vi "Umgebungsdruck beruecksichtigen.vi"(7 "CalGas":bool, 10 "Umgebungsdruck":sgl) -> (2 "Druck Sollwert":sgl)   [LabVIEW 2020, in "Regler.lvlib" / "Druckregler.lvlib"]
uses:
  Druckregler.lvlib
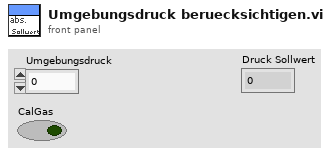
[diagram p1: front panel]
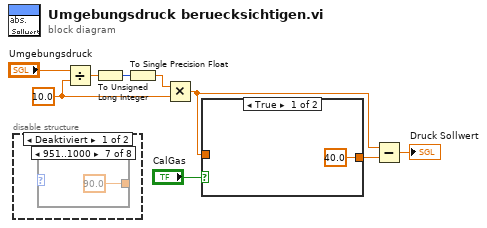
[diagram p0: block diagram]
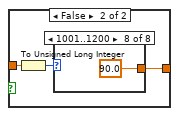
[diagram p2: hidden frame]
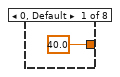
[diagram p3: hidden frame]
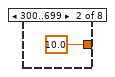
[diagram p4: hidden frame]
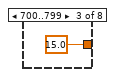
[diagram p5: hidden frame]
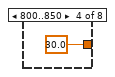
[diagram p6: hidden frame]
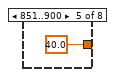
[diagram p7: hidden frame]
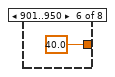
[diagram p8: hidden frame]
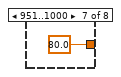
[diagram p9: hidden frame]
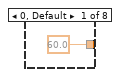
[diagram p10: hidden frame]
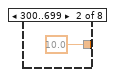
[diagram p11: hidden frame]
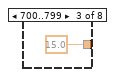
[diagram p12: hidden frame]
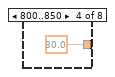
[diagram p13: hidden frame]
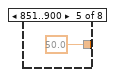
[diagram p14: hidden frame]
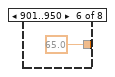
[diagram p15: hidden frame]
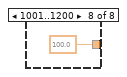
[diagram p16: hidden frame]
diagram:
  w5 = sgl 10.0 ("y")
  n1 = disable-structure shown="Deaktiviert" {
    frame Disabled {
      n2 = case shown="951..1000" {
        selector: _ -> [_ _ _ _ _ _ _ _]
        tunnel: [sgl 60.0 ("y") sgl 10.0 ("y") sgl 15.0 ("y") sgl 30.0 ("y") sgl 50.0 ("y") sgl 65.0 ("y") sgl 90.0 ("y") sgl 100.0 ("y")] -> _
        frame 0, Default {
        }
        frame 300..699 {
        }
        frame 700..799 {
        }
        frame 800..850 {
        }
        frame 851..900 {
        }
        frame 901..950 {
        }
        frame 951..1000 {
        }
        frame 1001..1200 {
        }
      }
    }
    frame Enabled {
    }
  }
  n3 = Divide(x="Umgebungsdruck", y=w5) -> (x/y=w8:sgl)
  n4 = To Unsigned Long Integer(number=w8) -> (unsigned 32bit integer=w7:u32)
  n5 = To Single Precision Float(number=w7) -> (single precision float=w6:sgl)
  n6 = Multiply(x=w6, y=w5) -> (x*y=w2:sgl)
  n7 = case shown="True" "CalGas" {
    tunnel: [sgl 40.0 ("y") w21] -> w9
    tunnel: w2 -> [_ w19]
    frame True {
    }
    frame False {
      n8 = To Unsigned Long Integer(number=w19) -> (unsigned 32bit integer=w20:u32)
      n9 = case shown="1001..1200" w20 {
        tunnel: [sgl 40.0 ("y") sgl 10.0 ("y") sgl 15.0 ("y") sgl 30.0 ("y") sgl 40.0 ("y") sgl 40.0 ("y") sgl 80.0 ("y") sgl 90.0 ("y")] -> w21
        frame 0, Default {
        }
        frame 300..699 {
        }
        frame 700..799 {
        }
        frame 800..850 {
        }
        frame 851..900 {
        }
        frame 901..950 {
        }
        frame 951..1000 {
        }
        frame 1001..1200 {
        }
      }
    }
  }
  n10 = Subtract(x=w2, y=w9) -> (x-y=→"Druck Sollwert":sgl)
